vi "Dequeue Log Entry.vi"(8 "error in (no error)":errorcluster, 9 "timeout in ms (-1)":i32=-1, 11 "Mock Log Handler in":refnum<class "Mock Log Handler.lvclass">) -> (0 "error out":errorcluster, 1 "timed out?":bool, 2 "Entry":T1, 3 "Mock Log Handler out":refnum<class "Mock Log Handler.lvclass">)   [LabVIEW 2020, in "Mock Log Handler.lvclass"]
uses:
  Mock Log Handler.lvclass
  Private/Log Entry.ctl
  Mock Log Handler.lvclass/Mock Log Handler.ctl
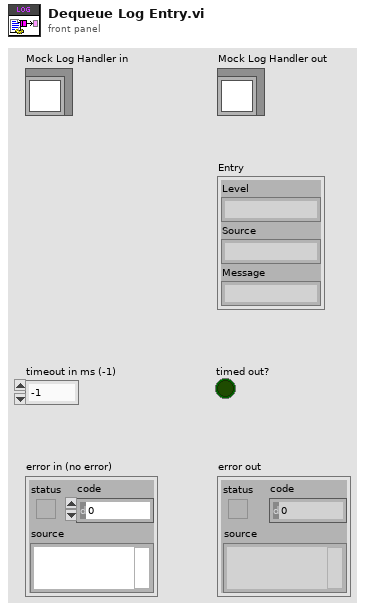
[diagram p1: front panel]
types:
  T1 = typedef "Mock Log Handler.lvclass/Log Entry.ctl" = cluster{"Level":string, "Source":string, "Message":string}
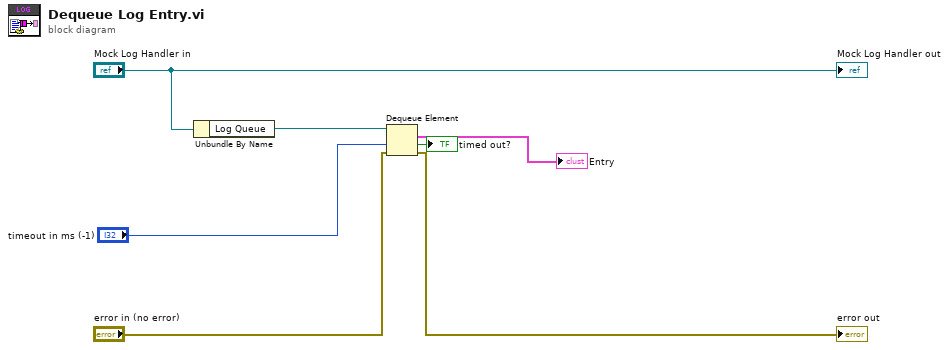
[diagram p0: block diagram]
diagram:
  n1 = Unbundle By Name("Mock Log Handler in") -> ("Log Queue"=w6:refnum<queue>)
  n2 = Dequeue Element(queue=w6, timeout in ms (-1)="timeout in ms (-1)", error in (no error)="error in (no error)") -> (element=→"Entry":T1, timed out?=→"timed out?":bool, error out=→"error out":errorcluster)  [unwired: 1 out]
  "Mock Log Handler out" <- "Mock Log Handler in"
